vi "Perform Work.vi"(6 "Last request":bool, 8 "error in (no error)":errorcluster, 9 "Initialize":bool, 10 "Reply to":refnum<class "Result Reply Msg.lvclass">, 11 "Measure Controller in":refnum<class "Process Controller.lvclass">) -> (0 "error out":errorcluster, 3 "Measure Controller out":refnum<class "Process Controller.lvclass">)   [LabVIEW 2018, in "Process Controller.lvclass"]
uses:
  Process Controller.lvclass
  C:/github/LabActor/Template Module/Template Module.lvclass
  Template Module Messages/Result Reply Msg/Result Reply Msg.lvclass
  Process Controller Messages/Result Response Msg/Result Response Msg.lvclass
  C:/github/LabActor/Template Module Messages/Result Reply Msg/Result Reply Msg.lvclass
  Template Module/Template Module.lvclass/Template Module.ctl
  Process Controller.lvclass/Process Controller.ctl
  NHMFL_Core/Libraries/Instruments/Results/Acquired Result/Acquired Result.lvclass
  Template Module Messages/Write tdms stream Msg/Write tdms stream Msg.lvclass/Write tdms stream Msg.ctl
  <vilib>/ActorFramework/Message Enqueuer/Message Enqueuer.lvclass/Message Enqueuer.ctl
  Worker Messages/Perform Work Msg/Perform Work Msg.lvclass/Perform Work Msg.ctl
  Template Module/Read Logger.vi
  <vilib>/ActorFramework/Message Enqueuer/Enqueue.vi
  Template Module Messages/Write tdms stream Msg/Write tdms stream Msg.lvclass
  C:/Program Files/National Instruments/LabVIEW 2018/vi.lib/ActorFramework/Message/Message.lvclass
  Worker Messages/Perform Work Msg/Perform Work Msg.lvclass
  <vilib>/ActorFramework/Message Priority Queue/Priority Enqueue.vi
  Loggers/Logger/Logger.lvclass
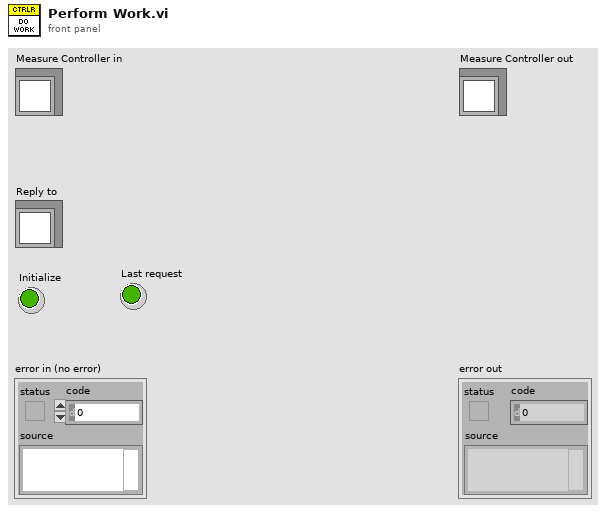
[diagram p1: front panel]
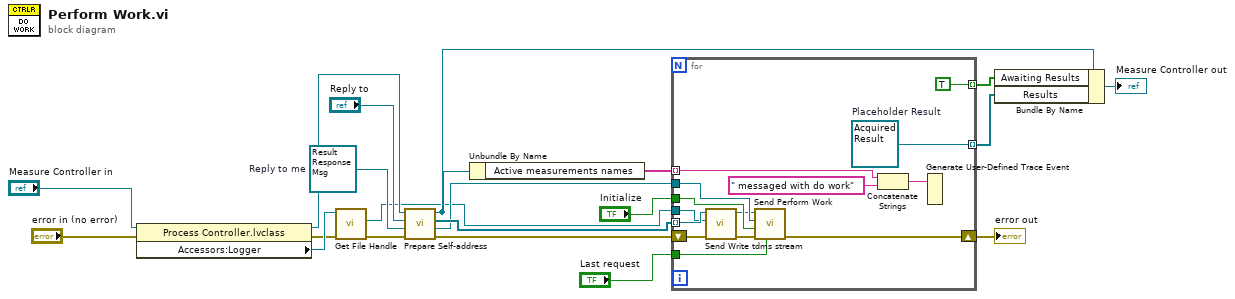
[diagram p0: block diagram]
diagram:
  w11 = refnum<class "Result Response Msg.lvclass"> refnum  # Reply to me
  n1 = property class="Process Controller.lvclass"(reference="Measure Controller in", error in="error in (no error)") -> (reference out=w10:refnum<class "Process Controller.lvclass">, error out=w2:errorcluster, "Accessors:Logger"=w9:refnum<class "Logger.lvclass">)
  n2 = call-dynamic "Get File Handle.vi"("error in (no error)"=w2, "Logger in"=w9) -> ("error out"=w1:errorcluster, "File handle"=w3:refnum<k34>)  [unwired: 5 in, 3 out]
  n3 = call-dynamic "Prepare Self-address.vi"("error in (no error)"=w1, "Reply to me"=w11, "Reply to"="Reply to", "Process Controller in"=w10) -> ("error out"=w7:errorcluster, "Reply to me"=w12:refnum<class "Result Reply Msg.lvclass">, "Active measurements enqueuers"=w13:refnum<class "Message Enqueuer.lvclass">[], "Process Controller out"=w5:refnum<class "Process Controller.lvclass">)  [unwired: 4 in]
  n4 = Unbundle By Name(w5) -> ("Active measurements names"=w4:string[])
  n5 = for {
    shift-right: [w34] -> w17
    shift-left: w7 -> [w27]
    tunnel: "Initialize" -> [w31]
    tunnel: [TRUE] -> w20 mode=indexing
    tunnel: [w32] -> w19 mode=indexing
    tunnel: w13 -> [w29] mode=indexing
    tunnel: w12 -> [w30]
    tunnel: w3 -> [w25]
    tunnel: "Last request" -> [w24]
    tunnel: w4 -> [w21] mode=indexing
    w32 = refnum<class "Acquired Result.lvclass"> refnum  # Placeholder Result
    n6 = call "Send Write tdms stream.vi"("error in (no error)"=w27, "tdms stream"=w25, "Message Enqueuer"=w29) -> ("error out"=w26:errorcluster, "Message Enqueuer out"=w28:refnum<class "Message Enqueuer.lvclass">)  [unwired: 7 in]
    n7 = call "Send Perform Work.vi"("Last request"=w24, "error in (no error)"=w26, "Initialize"=w31, "Reply to"=w30, "Message Enqueuer"=w28) -> ("error out"=w34:errorcluster)  [unwired: 5 in, 1 out]
    n8 = Concatenate Strings(w21, " messaged with do work" ("string")) -> (w23:string)
    n9 = Generate User-Defined Trace Event(2:w23) -> ()  [unwired: 1 in]
  }
  "error out" <- w17
  n10 = Bundle By Name(cluster=w5, "Awaiting Results"=w20, "Results"=w19) -> (→"Measure Controller out":refnum<class "Process Controller.lvclass">)
